vi "GetDeviceIdentificationSCPI.vi"(8 "error in":errorcluster, 11 "VISA resource name":refnum<visa-resource-name>) -> (0 "error out":errorcluster, 2 "8800 Response Identification":string, 3 "VISA resource name out":refnum<visa-resource-name>)   [LabVIEW 2023, in "Thermotron 8800.lvlib"]
doc: "*IDN?\nCommand name: SCPI-compatible device identification\nCommand type: System status\nDescription: Manufacturer, chamber description:controller model, chamber serial number, firmware\nrevision\nSyntax: *IDN?\nData type: ASCII character string\nQuery example: *IDN?\n8800 response: Thermotron Industries, 8800 Chamber Controller:8800, 45194, V4.71"
uses:
  Thermotron 8800.lvlib
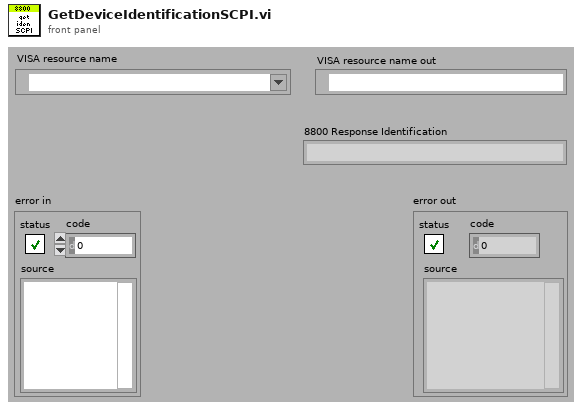
[diagram p1: front panel]
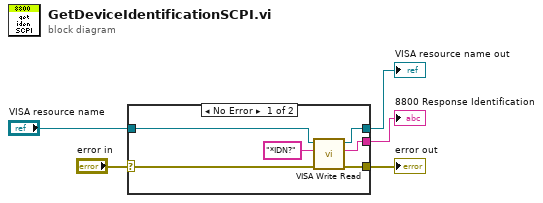
[diagram p0: block diagram]
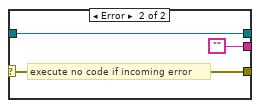
[diagram p2: hidden frame]
diagram:
  n1 = case shown="No Error" "error in" {
    selector: "error in" -> [w11 w14]
    tunnel: [w9 w14] -> w1
    tunnel: [w10 w12] -> w4
    tunnel: [w8 ""] -> w5
    tunnel: "VISA resource name" -> [w7 w12]
    frame No Error {
      n2 = call "VISA Write Read.vi"("error in (no error)"=w11, "8800 Command"="*IDN?", "VISA Refnum in"=w7) -> ("error out"=w9:errorcluster, "read buffer"=w8:string, "VISA Refnum out"=w10:refnum<visa-resource-name>)  [unwired: 6 in]
    }
    frame Error {
      # "execute no code if incoming error"
    }
  }
  "VISA resource name out" <- w4
  "error out" <- w1
  "8800 Response Identification" <- w5
